vi "Destroy Server.vi"(8 "error in (no error)":errorcluster, 11 "Server in":refnum<class "Server.lvclass">) -> (0 "error out":errorcluster, 3 "Server out":refnum<class "Server.lvclass">)   [LabVIEW 2013, in "MQTT Server.lvlib" / "Server.lvclass"]
uses:
  Server.lvclass
  Server.lvclass/Server.ctl
  StoredSessions/StoredSessions.lvclass
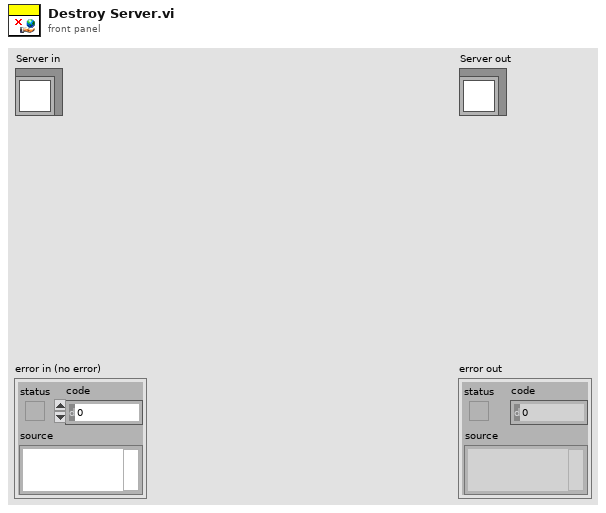
[diagram p1: front panel]
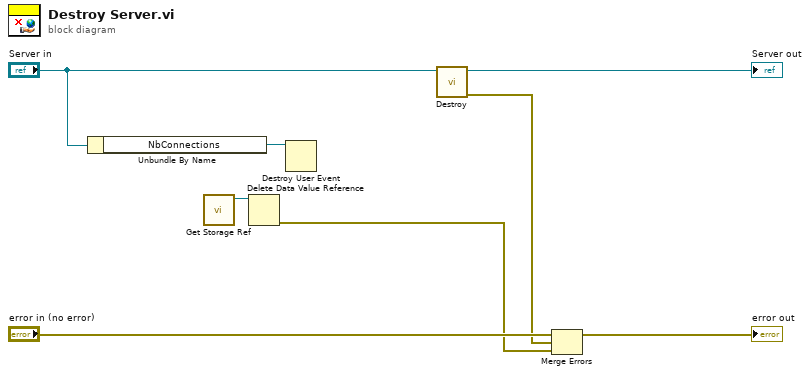
[diagram p0: block diagram]
diagram:
  n1 = Unbundle By Name("Server in") -> ("NbConnections"=w4:refnum<user-event>)
  n2 = call "Get Storage Ref.vi"() -> ("Storage"=w6:refnum<data-value>)  [unwired: 11 in]
  n3 = Delete Data Value Reference(data value reference=w6) -> (error out=w5:errorcluster)  [unwired: 1 in, 1 out]
  n4 = Destroy User Event(user event=w4) -> ()  [unwired: 1 in, 1 out]
  n5 = call-dynamic "Destroy.vi"("MQTT_Base in"="Server in") -> ("error out"=w1:errorcluster, "MQTT_Base out"=→"Server out":refnum<class "Server.lvclass">)  [unwired: 9 in]
  n6 = Merge Errors("error in (no error)", w1, w5) -> (→"error out":errorcluster)
